vi "BPSK_Modulation.vi"(5 "EN_Modulation":dbl, 8 "error in (no error)":errorcluster caption="错误输入（无错误）", 10 "input_data":dbl[](array[numeric]) format="%#_13g", 11 "PathIn":path) -> (0 "error out":errorcluster caption="错误输出", 3 "PathOut":path, 6 "output_data":dbl[](array[numeric]), 7 "y":dbl[](array[numeric]))   [LabVIEW 2015]
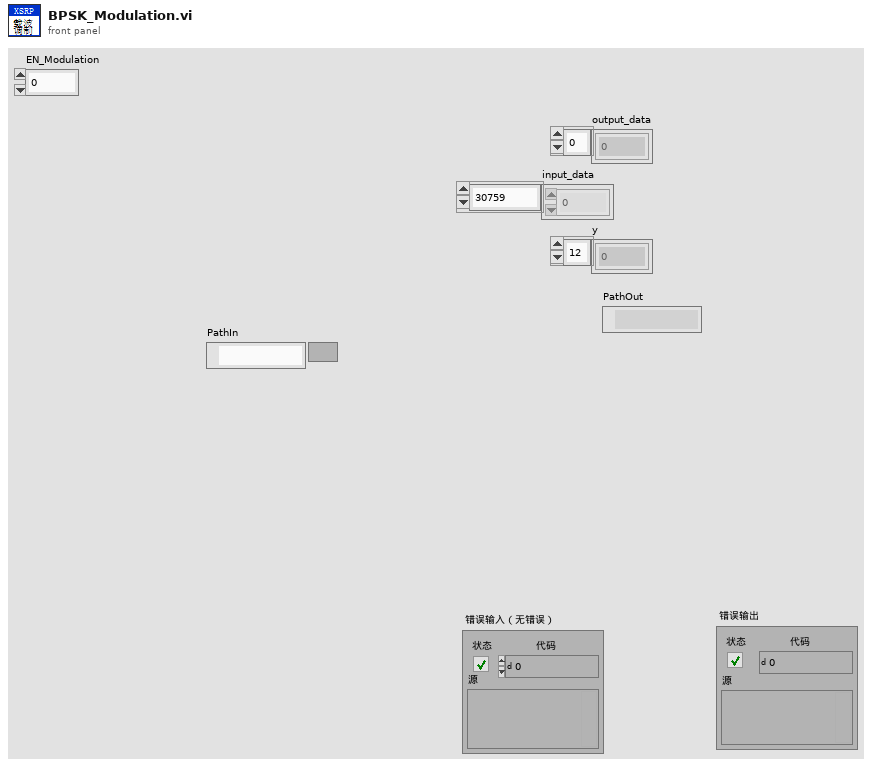
[diagram p1: front panel]
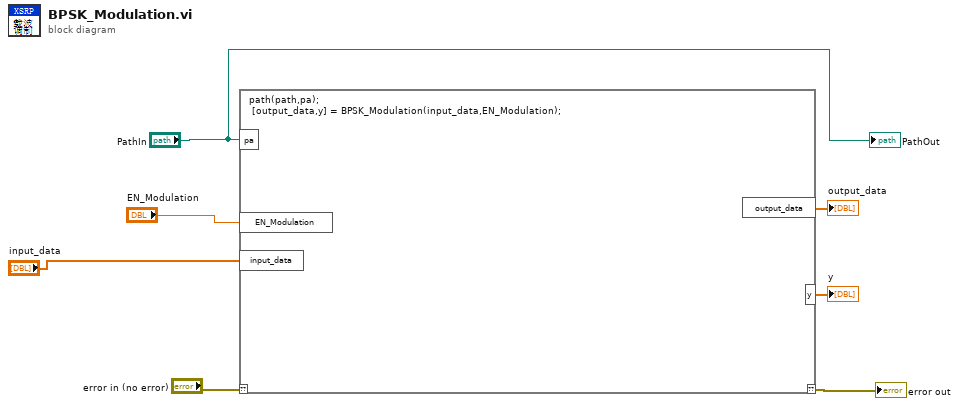
[diagram p0: block diagram]
diagram:
  n1 = script code="path(path,pa);\n [output_data,y] = BPSK_Modulation(input_data,EN_Modulation);"("??"="error in (no error)", "pa"="PathIn", "input_data"="input_data", "EN_Modulation"="EN_Modulation") -> ("??"=→"error out":errorcluster, "y"=→"y":dbl[], "output_data"=→"output_data":dbl[])
  "PathOut" <- "PathIn"
